vi "Flush Win Msg Q.vi"(4 "error in (no error)":errorcluster, 7 "win msg queue":T1) -> (0 "error out":errorcluster, 3 "win msg queue out":T1)   [LabVIEW 2011]
doc: "Removes all pending windows messages in the windows message queue.\n\nParameters:\nwin msg queue: the queue whose elements should be deleted.\n\nErrors:\nReturns 6751 if win msg queue is not a valid windows message queue."
uses:
  Win Msg Q RefNum.ctl
  lvwinmsg.dll
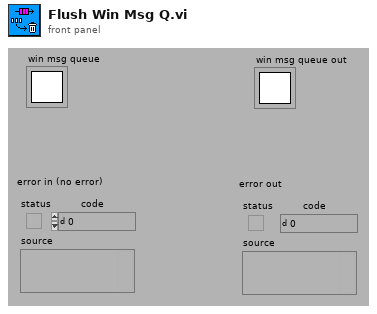
[diagram p1: front panel]
types:
  T1 = typedef "Win Msg Q RefNum.ctl" = refnum<k1>
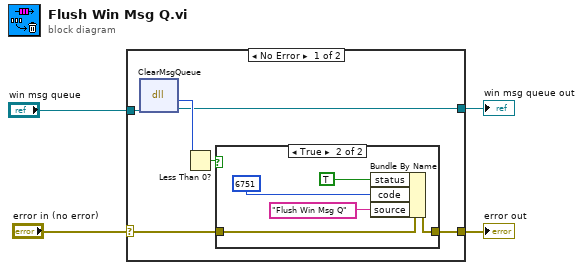
[diagram p0: block diagram]
diagram:
  n1 = case shown="No Error" "error in (no error)" {
    selector: "error in (no error)" -> [w5 w17]
    tunnel: "win msg queue" -> [w8 w18]
    tunnel: [w9 w17] -> w3
    tunnel: [w6 w18] -> w2
    frame No Error {
      n2 = dll-call lib="C:/Development/SI.LIB/WIN32/WinMSGQ/lvwinmsg.dll" fn="ClearMsgQueue"("win msg queue"=w8) -> (w7:i32, "win msg queue"=w6:T1)  [unwired: 3 in, 2 out]
      n3 = Less Than 0?(x=w7) -> (x < 0?=w10:bool)
      n4 = case shown="True" w10 {
        tunnel: w5 -> [w11 w14]
        tunnel: [w11 w13] -> w9
        frame False {
        }
        frame True {
          n5 = Bundle By Name(cluster=w14, "status"=TRUE, "code"=6751 ("Error Code"), "source"="Flush Win Msg Q") -> (w13:errorcluster)
        }
      }
    }
    frame Error {
    }
  }
  "error out" <- w3
  "win msg queue out" <- w2
